vi "Bundle Script_Named (Un)Bundler Move Up or Down.vi"(7 "Action":T1(ring)=enum."Wire Properties", 10 "index":u16, 11 "Elements Array":T2(array[cluster])) -> ()   [LabVIEW 2023]
panel:
  out "Elements Array 2":T2(array[cluster])
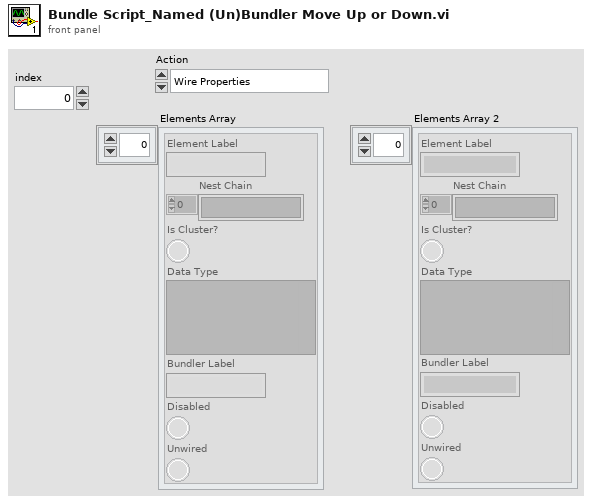
[diagram p1: front panel]
types:
  T1 = enum16{"[NONE]", "Wire Bundle", "Wire Unbundle", "Terminal Unbundle", "Terminal Bundle", "Bundler Move Up", "Bundler Move Down", "Bundler Insert", "Bundler Remove", "Bundler Remove Unwired", "Bundler Rearrange", "In Place Insert", "In Place Remove", "In Place Remove Unwired", "In Place Rearrange", "Wire Properties", "Wire Method", "Terminal Properties", "Terminal Method", "Property Move Up", "Property Move Down", "Properties Insert", "Properties Remove", "Properties Remove Unwired", "Properties Rearrange", "Method Change", "Class for Constant", "Class For Control", "Class For Node", "Class Name to Clipboard"}
  T2 = cluster{"Element Label":string, "Nest Chain":string[], "Is Cluster?":bool, "Data Type":variant, "Bundler Label":string, "Disabled":bool, "Unwired":bool}[]
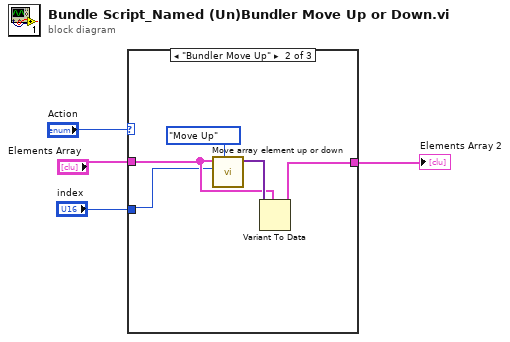
[diagram p0: block diagram]
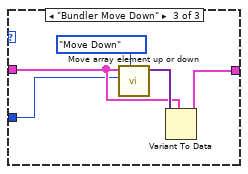
[diagram p3: hidden frame]
diagram:
  n1 = case shown="\"Bundler Move Up\"" "Action" {
    tunnel: "Elements Array" -> [w5 w8 w13]
    tunnel: [w5 w7 w12] -> w2
    tunnel: "index" -> [_ w6 w11]
    frame "[NONE]", Default {
    }
    frame "Bundler Move Up" {
      n2 = call "Move array element up or down.vi"("Action"=enum16{"Move Up", "Move Down"}."Move Up", "index"=w6, "Array In"=w8) -> ("Array Out"=w10:variant[])  [unwired: 8 in]
      n3 = Variant To Data(type=w8, Variant=w10) -> (data=w7:T2)  [unwired: 1 in, 1 out]
    }
    frame "Bundler Move Down" {
      n4 = call "Move array element up or down.vi"("Action"=enum16{"Move Up", "Move Down"}."Move Down", "index"=w11, "Array In"=w13) -> ("Array Out"=w14:variant[])  [unwired: 8 in]
      n5 = Variant To Data(type=w13, Variant=w14) -> (data=w12:T2)  [unwired: 1 in, 1 out]
    }
  }
  "Elements Array 2" <- w2
